vi "Testing Gluing Motion.vi"() -> ()   [LabVIEW 2011]
uses:
  UI typedefs/BBM Chuck Used.ctl
  UI typedefs/Glue Paths.ctl
  UI typedefs/Glue Path.ctl
  Shared Components/WorkTable Class/Type Definitions/Worktable_Mode.ctl
  Shared Components/Gantry Class/Gantry Class.lvclass
  Shared Components/GrabberTool Class/GrabberTool Class.lvclass
  Shared Components/WorkTable Class/WorkTable Class.lvclass
  Shared Components/PickerTool Class/PickerTool Class.lvclass
panel:
  in  "Glue Pathways":T1 {"BBM Slot" items=["Slot 1", "Slot 2", "Slot 3", "Slot 4"]; "Weight Slot" items=["Slot 1", "Slot 2", "Slot 3", "Slot 4"]; "Glue Slot" items=["Slot 1", "Slot 2", "Slot 3", "Slot 4"]; "Stamp Slot" items=["Slot 1", "Slot 2", "Slot 3", "Slot 4"]; "HDI Slot" items=["Slot 1", "Slot 2", "Slot 3", "Slot 4"]}
  in  "Config Folder":path=path "C:/Users/husker/Desktop/gantry/Config"
  in  "Virtual Mode":bool
  in  "Which Path?":i32
  out "error out":errorcluster
  in  "Chuck Module Used for BBM:":T3 items=["Chuck 1", "Chuck 2", "Chuck 3", "Chuck 4"]
  in  "Active Path (0-3)":bool[](array[boolean])
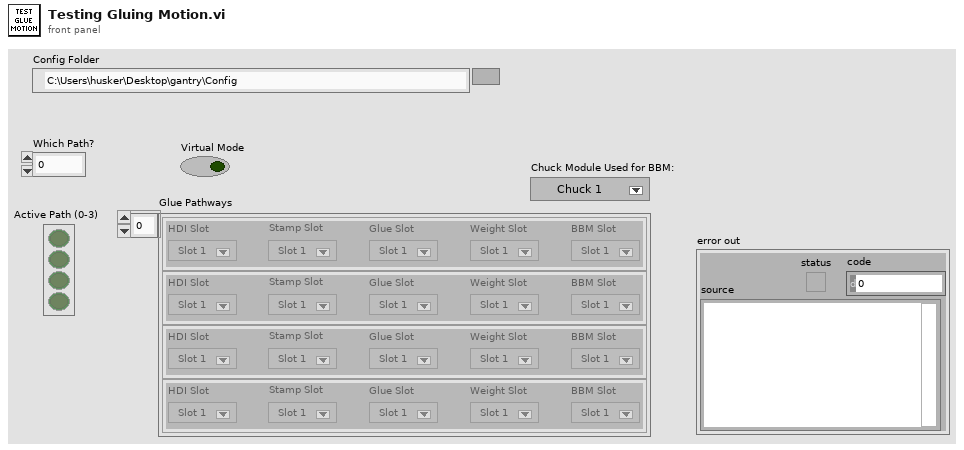
[diagram p1: front panel]
types:
  T1 = typedef "Glue Paths.ctl" = T2[]
  T2 = typedef "Glue Path.ctl" = cluster{"HDI Slot ":i32, "Stamp Slot":i32, "Glue Slot":i32, "Weight Slot":i32, "BBM Slot":i32}
  T3 = typedef "BBM Chuck Used.ctl" = i32
  T4 = typedef "Worktable_Mode.ctl" = enum16{"Encapsulation", "Gluing"}
  T5 = enum16{"Empty", "Bare HDI", "Unglued", "Stamped", "PartOnTop", "Weighted", "Unpotted", "Potted"}
  T6 = typedef "Worktable_Stamp.ctl" = cluster{"Stamp State":enum16{"Empty", "Populated", "Used"}, "Location/Orientation":T7, "Stamp Type":T8}
  T7 = typedef "Position_Orientation.ctl" = cluster{"Center":refnum<class "Vec3d Class.lvclass">, "Orientation":refnum<class "Orient3d Class.lvclass">}
  T8 = typedef "Stamp Type.ctl" = enum16{"Stamp 1", "Stamp 2", "Stamp 3", "Stamp 4", "Stamp 5"}
  T9 = cluster{"Reservoir State":enum16{"Empty", "Full", "Used"}, "Center":refnum<class "Vec3d Class.lvclass">}
  T10 = typedef "Worktable_Module Slot.ctl" = cluster{"Slot State":enum16{"Empty", "Bare HDI", "Unglued", "Stamped", "PartOnTop", "Weighted", "Unpotted", "Potted"}, "BBM Type":enum16{"None", "BBM", "GlassSlide"}, "HDI Type":enum16{"None", "HDI", "Polyimide"}, "Vacuum Channel":u8, "Location/Orientation BBM":T7, "Location/Orientation HDI":T7, "S/N":string}
  T11 = typedef "Worktable_Weight.ctl" = cluster{"Weight State":enum16{"Empty", "Populated"}, "Weight Type":T12, "Location/Orientation":T7}
  T12 = typedef "Weight Type.ctl" = enum16{"Weight 1", "Weight 2", "Weight 3", "Weight 4", "Weight 5", "Weight 6", "Weight 7", "Weight 8"}
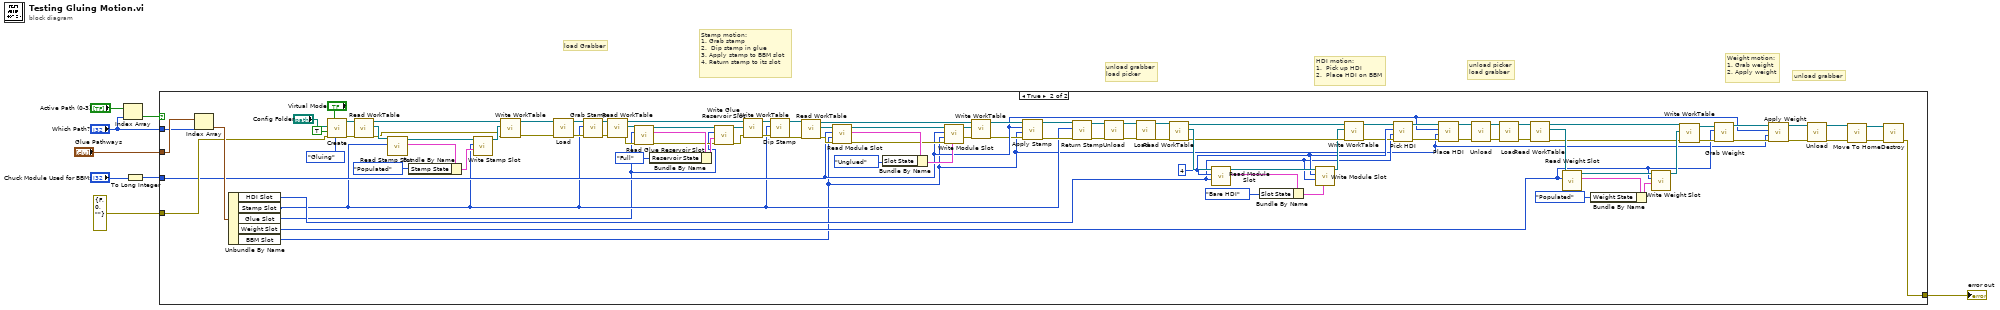
[diagram p0: block diagram]
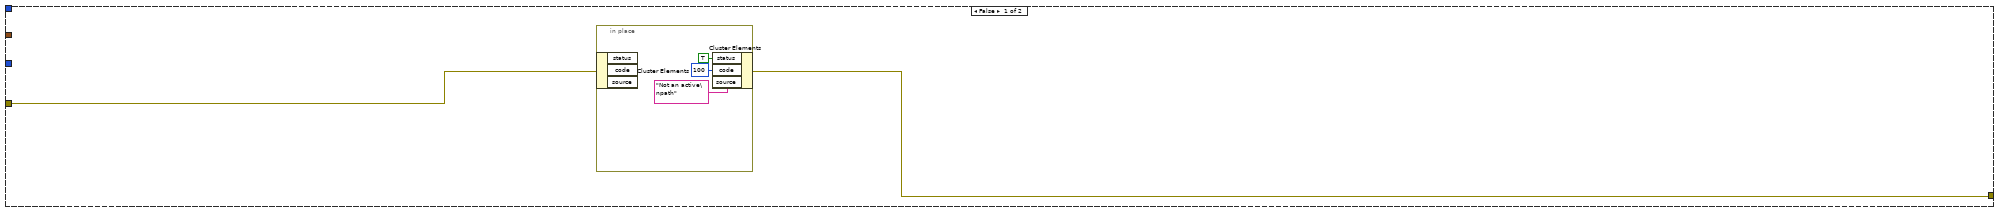
[diagram p2: hidden frame]
diagram:
  # "unload grabber"
  # "unload picker\nload grabber"
  # "unload grabber\nload picker"
  # "load Grabber"
  # "Weight motion:\n1. Grab weight\n2. Apply weight"
  # "HDI motion:\n1.  Pick up HDI\n2.  Place HDI on BBM"
  # "Stamp motion:\n1. Grab stamp\n2.  Dip stamp in glue\n3. Apply stamp to BBM slot\n4. Return stamp to its slot"
  n1 = Index Array(array="Active Path (0-3)", index="Which Path?") -> (element=w7:bool)
  n2 = To Long Integer(number="Chuck Module Used for BBM:") -> (32bit integer=w2:T3)
  n3 = case shown="True" w7 {
    tunnel: "Glue Pathways" -> [_ w114]
    tunnel: "Which Path?" -> [_ w113]
    tunnel: errorcluster {"status"=FALSE, "code"=0, "source"=""} ("error constant") -> [w10 w63]
    tunnel: [w9 w41] -> w5
    tunnel: w2 -> [_ w46]
    frame False {
      n4 = in-place {
        n5 = in-place-cluster #1(w10) -> ()  [unwired: 3 out]
        n6 = in-place-cluster #1("status"=TRUE, "code"=100, "source"="Not an active\npath") -> (w9:errorcluster)
      }
    }
    frame True {
      w60 = 4 ("chuck")
      n7 = Index Array(array=w114, index=w113) -> (element=w115:T2)
      n8 = Unbundle By Name(w115) -> ("HDI Slot"=w18:i32, "Stamp Slot"=w17:i32, "Glue Slot"=w16:i32, "Weight Slot"=w15:i32, "BBM Slot"=w14:i32)
      n9 = call "Create.vi"("Worktable Mode"=Worktable_Mode."Gluing", "Virtual Mode"="Virtual Mode", "error in"=w63, "HOME?"=TRUE, "Config Folder"="Config Folder") -> ("error out"=w19:errorcluster, "Gantry out"=w112:refnum<class "Gantry Class.lvclass">)  [unwired: 5 in]
      n10 = call-dynamic "Read WorkTable.vi"("error in"=w19, "Gantry Class in"=w112) -> ("error out"=w20:errorcluster, "WorkTable Class.lvclass"=w111:refnum<class "WorkTable Class.lvclass">, "Gantry Class out"=w105:refnum<class "Gantry Class.lvclass">)  [unwired: 7 in]
      n11 = call "Read Stamp Slot.vi"("Stamp Slot"=w17, "WorkTable Class in"=w111) -> ("Stamp Slot"=w110:T6, "WorkTable Class out"=w107:refnum<class "WorkTable Class.lvclass">)  [unwired: 7 in, 1 out]
      n12 = Bundle By Name(cluster=w110, "Stamp State"=enum16{"Empty", "Populated", "Used"}."Populated") -> (w108:T6)
      n13 = call "Write Stamp Slot.vi"(9:"Stamp Slot"=w108, 10:"Stamp Slot"=w17, "WorkTable Class in"=w107) -> ("WorkTable Class out"=w106:refnum<class "WorkTable Class.lvclass">)  [unwired: 7 in, 1 out]
      n14 = call-dynamic "Write WorkTable.vi"("error in (no error)"=w20, "WorkTable Class.lvclass"=w106, "Gantry Class in"=w105) -> ("error out"=w21:errorcluster, "Gantry Class out"=w104:refnum<class "Gantry Class.lvclass">)  [unwired: 7 in]
      n15 = call "Load.vi"("error in"=w21, "Gantry In"=w104) -> ("error out"=w22:errorcluster, "Grabber Tool out"=w103:refnum<class "GrabberTool Class.lvclass">)  [unwired: 8 in]
      n16 = call "Grab Stamp.vi"("error in"=w22, "Stamp Number"=w17, "GrabberTool in"=w103) -> ("error out"=w23:errorcluster, "GrabberTool out"=w92:refnum<class "GrabberTool Class.lvclass">)  [unwired: 7 in]
      n17 = call-dynamic "Read WorkTable.vi"("error in"=w23, "Gantry Class in"=w92) -> ("error out"=w101:errorcluster, "WorkTable Class.lvclass"=w102:refnum<class "WorkTable Class.lvclass">, "Gantry Class out"=w95:refnum<class "GrabberTool Class.lvclass">)  [unwired: 7 in]
      n18 = call "Read Glue Reservoir Slot.vi"("error in (no error)"=w101, "index"=w16, "WorkTable Class in"=w102) -> ("error out"=w97:errorcluster, "Glue Resivoir Slot"=w100:T9, "WorkTable Class out"=w96:refnum<class "WorkTable Class.lvclass">)  [unwired: 6 in]
      n19 = Bundle By Name(cluster=w100, "Reservoir State"=enum16{"Empty", "Full", "Used"}."Full") -> (w98:T9)
      n20 = call "Write Glue Reservoir Slot.vi"("error in (no error)"=w97, "Glue Resivoir Slot"=w98, "index"=w16, "WorkTable Class in"=w96) -> ("error out"=w93:errorcluster, "WorkTable Class out"=w94:refnum<class "WorkTable Class.lvclass">)  [unwired: 6 in]
      n21 = call-dynamic "Write WorkTable.vi"("error in (no error)"=w93, "WorkTable Class.lvclass"=w94, "Gantry Class in"=w95) -> ("error out"=w24:errorcluster, "Gantry Class out"=w91:refnum<class "GrabberTool Class.lvclass">)  [unwired: 7 in]
      n22 = call "Dip Stamp.vi"("error in"=w24, "Reservoir Number"=w17, "GrabberTool in"=w91) -> ("error out"=w25:errorcluster, "GrabberTool out"=w80:refnum<class "GrabberTool Class.lvclass">)  [unwired: 7 in]
      n23 = call-dynamic "Read WorkTable.vi"("error in"=w25, "Gantry Class in"=w80) -> ("error out"=w89:errorcluster, "WorkTable Class.lvclass"=w90:refnum<class "WorkTable Class.lvclass">, "Gantry Class out"=w85:refnum<class "GrabberTool Class.lvclass">)  [unwired: 7 in]
      n24 = call-dynamic "Read Module Slot.vi"("error in"=w89, "slot"=w14, "chuck"=w46, "WorkTable in"=w90) -> ("error out"=w86:errorcluster, "Module Slot"=w88:T10, "WorkTable out"=w84:refnum<class "WorkTable Class.lvclass">)  [unwired: 5 in]
      n25 = Bundle By Name(cluster=w88, "Slot State"=T5."Unglued") -> (w87:T10)
      n26 = call-dynamic "Write Module Slot.vi"("Module Slot"=w87, "error in"=w86, "slot"=w14, "chuck"=w46, "WorkTable in"=w84) -> ("error out"=w82:errorcluster, "WorkTable out"=w83:refnum<class "WorkTable Class.lvclass">)  [unwired: 5 in]
      n27 = call-dynamic "Write WorkTable.vi"("error in (no error)"=w82, "WorkTable Class.lvclass"=w83, "Gantry Class in"=w85) -> ("error out"=w26:errorcluster, "Gantry Class out"=w79:refnum<class "GrabberTool Class.lvclass">)  [unwired: 7 in]
      n28 = call "Apply Stamp.vi"("error in"=w26, "Slot Number"=w14, "Chuck Number"=w46, "GrabberTool in"=w79) -> ("error out"=w27:errorcluster, "GrabberTool out"=w78:refnum<class "GrabberTool Class.lvclass">)  [unwired: 6 in]
      n29 = call "Return Stamp.vi"("error in"=w27, "Slot Number"=w17, "GrabberTool in"=w78) -> ("error out"=w28:errorcluster, "GrabberTool out"=w77:refnum<class "GrabberTool Class.lvclass">)  [unwired: 7 in]
      n30 = call "Unload.vi"("error in"=w28, "GrabberTool in"=w77) -> ("error out"=w29:errorcluster, "Gantry out"=w76:refnum<class "Gantry Class.lvclass">)  [unwired: 8 in]
      n31 = call "Load.vi"("error in"=w29, "Gantry in"=w76) -> ("error out"=w30:errorcluster, "PickerTool out"=w67:refnum<class "PickerTool Class.lvclass">)  [unwired: 8 in]
      n32 = call-dynamic "Read WorkTable.vi"("error in"=w30, "Gantry Class in"=w67) -> ("error out"=w69:errorcluster, "WorkTable Class.lvclass"=w71:refnum<class "WorkTable Class.lvclass">, "Gantry Class out"=w70:refnum<class "PickerTool Class.lvclass">)  [unwired: 7 in]
      n33 = call-dynamic "Read Module Slot.vi"("slot"=w18, "chuck"=w60, "WorkTable in"=w71) -> ("Module Slot"=w75:T10, "WorkTable out"=w72:refnum<class "WorkTable Class.lvclass">)  [unwired: 6 in, 1 out]
      n34 = Bundle By Name(cluster=w75, "Slot State"=T5."Bare HDI") -> (w73:T10)
      n35 = call-dynamic "Write Module Slot.vi"("Module Slot"=w73, "slot"=w18, "chuck"=w60, "WorkTable in"=w72) -> ("WorkTable out"=w68:refnum<class "WorkTable Class.lvclass">)  [unwired: 6 in, 1 out]
      n36 = call-dynamic "Write WorkTable.vi"("error in (no error)"=w69, "WorkTable Class.lvclass"=w68, "Gantry Class in"=w70) -> ("error out"=w31:errorcluster, "Gantry Class out"=w61:refnum<class "PickerTool Class.lvclass">)  [unwired: 7 in]
      n37 = call-dynamic "Pick HDI.vi"("error in"=w31, "Slot"=w18, "Chuck"=w60, "PickerTool in"=w61) -> ("error out"=w32:errorcluster, "PickerTool out"=w59:refnum<class "PickerTool Class.lvclass">)  [unwired: 6 in]
      n38 = call-dynamic "Place HDI.vi"("error in"=w32, "Slot Number"=w14, "Chuck Number"=w46, "PickupTool in"=w59) -> ("error out"=w33:errorcluster, "PickupTool out"=w58:refnum<class "PickerTool Class.lvclass">)  [unwired: 6 in]
      n39 = call "Unload.vi"("error in"=w33, "PickupTool in"=w58) -> ("error out"=w34:errorcluster, "Gantry out"=w57:refnum<class "Gantry Class.lvclass">)  [unwired: 8 in]
      n40 = call "Load.vi"("error in"=w34, "Gantry In"=w57) -> ("error out"=w35:errorcluster, "Grabber Tool out"=w56:refnum<class "GrabberTool Class.lvclass">)  [unwired: 8 in]
      n41 = call-dynamic "Read WorkTable.vi"("error in"=w35, "Gantry Class in"=w56) -> ("error out"=w36:errorcluster, "WorkTable Class.lvclass"=w55:refnum<class "WorkTable Class.lvclass">, "Gantry Class out"=w49:refnum<class "GrabberTool Class.lvclass">)  [unwired: 7 in]
      n42 = call "Read Weight Slot.vi"("weight slot"=w15, "WorkTable Class in"=w55) -> ("Weight Slot"=w54:T11, "WorkTable Class out"=w51:refnum<class "WorkTable Class.lvclass">)  [unwired: 7 in, 1 out]
      n43 = Bundle By Name(cluster=w54, "Weight State"=enum16{"Empty", "Populated"}."Populated") -> (w52:T11)
      n44 = call "Write Weight Slot.vi"("Weight Slot"=w52, "weight slot"=w15, "WorkTable Class in"=w51) -> ("WorkTable Class out"=w50:refnum<class "WorkTable Class.lvclass">)  [unwired: 7 in, 1 out]
      n45 = call-dynamic "Write WorkTable.vi"("error in (no error)"=w36, "WorkTable Class.lvclass"=w50, "Gantry Class in"=w49) -> ("error out"=w37:errorcluster, "Gantry Class out"=w48:refnum<class "GrabberTool Class.lvclass">)  [unwired: 7 in]
      n46 = call "Grab Weight.vi"("error in"=w37, "Weight Number"=w15, "GrabberTool in"=w48) -> ("error out"=w38:errorcluster, "GrabberTool out"=w47:refnum<class "GrabberTool Class.lvclass">)  [unwired: 7 in]
      n47 = call "Apply Weight.vi"("error in"=w38, "Slot Number"=w14, "Chuck Number"=w46, "GrabberTool in"=w47) -> ("error out"=w39:errorcluster, "GrabberTool out"=w45:refnum<class "GrabberTool Class.lvclass">)  [unwired: 6 in]
      n48 = call "Unload.vi"("error in"=w39, "GrabberTool in"=w45) -> ("error out"=w40:errorcluster, "Gantry out"=w42:refnum<class "Gantry Class.lvclass">)  [unwired: 8 in]
      n49 = call-dynamic "Move To Home.vi"("error in"=w40, "Gantry in"=w42) -> ("error out"=w44:errorcluster, "Gantry out"=w43:refnum<class "Gantry Class.lvclass">)  [unwired: 8 in]
      n50 = call "Destroy.vi"("error in"=w44, "Gantry Class in"=w43) -> ("error out"=w41:errorcluster)  [unwired: 9 in]
    }
  }
  "error out" <- w5
